vi "Query Output.vi"(8 "error in (no error)":errorcluster, 11 "FunctionGenerator in":refnum<class "FunctionGenerator.lvclass">) -> (0 "error out":errorcluster, 2 "Output":bool, 3 "FunctionGenerator out":refnum<class "FunctionGenerator.lvclass">)   [LabVIEW 2019, in "FunctionGenerator.lvlib" / "FunctionGenerator.lvclass"]
uses:
  Library/FunctionGenerator.lvclass
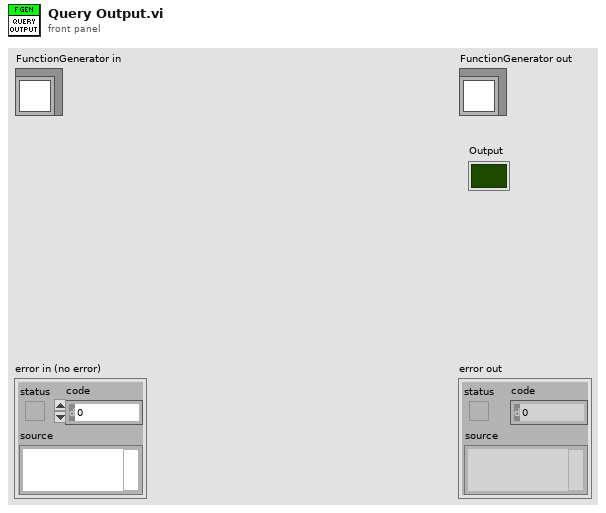
[diagram p1: front panel]
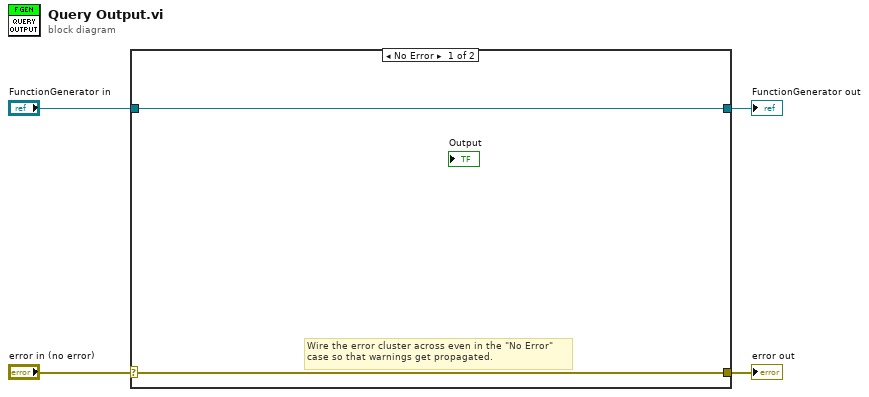
[diagram p0: block diagram]
diagram:
  n1 = case shown="No Error" "error in (no error)" {
    selector: "error in (no error)" -> [w5 w8]
    tunnel: [w5 w8] -> w3
    tunnel: [w6 w7] -> w1
    tunnel: "FunctionGenerator in" -> [w6 w7]
    frame No Error {
      # "Wire the error cluster across even in the \"No Error\"\ncase so that warnings get propagated."
    }
    frame Error {
    }
  }
  "error out" <- w3
  "FunctionGenerator out" <- w1
